vi "Determine Platform.vi"(8 "error in (no error)":errorcluster) -> (0 "error out":errorcluster, 3 "Platform":T1)   [LabVIEW 2020, in "binary_installation_tools.lvlib"]
uses:
  binary_installation_tools.lvlib
  Binary Dependency Platform.ctl
  <vilib>/Utility/error.llb/Clear Errors.vi
  <vilib>/Platform/system.llb/System Exec.vi
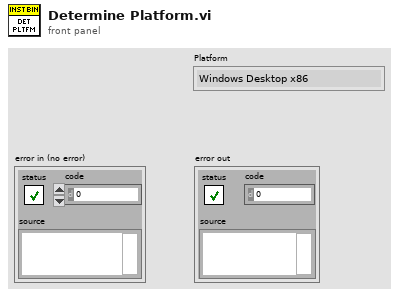
[diagram p1: front panel]
types:
  T1 = typedef "binary_installation_tools.lvlib/Binary Dependency Platform.ctl" = enum16{"Windows Desktop x86", "Windows Desktop x64", "Linux Desktop x64", "Linux Desktop aarch64", "NI Linux RT x64", "NI Linux RT armv7a"}
  T2 = typedef "binary_installation_tools.lvlib/Processor Architecture.ctl" = enum16{"Unknown", "x86", "x64", "arm", "arm64"}
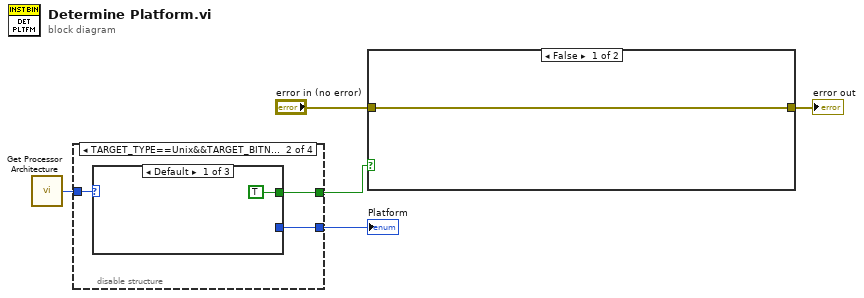
[diagram p0: block diagram]
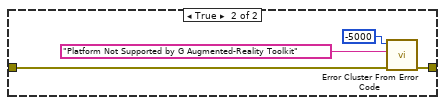
[diagram p2: hidden frame]
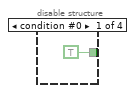
[diagram p3: hidden frame]
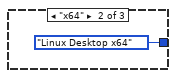
[diagram p4: hidden frame]
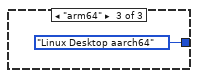
[diagram p5: hidden frame]
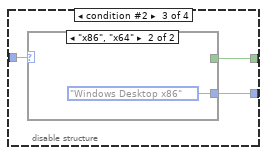
[diagram p6: hidden frame]
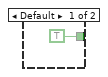
[diagram p7: hidden frame]
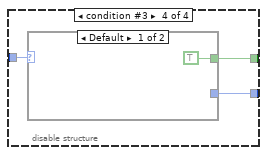
[diagram p8: hidden frame]
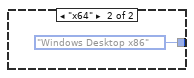
[diagram p9: hidden frame]
diagram:
  n1 = call "Get Processor Architecture.vi"() -> ("Processor Architecture"=w1:T2)
  n2 = disable-structure shown="TARGET_TYPE==Unix&&TARGET_BITNESS==64" {
    disable-tunnel: [_ w9 w15 w20] -> w5
    disable-tunnel: [TRUE w7 w13 w18] -> w2
    disable-tunnel: w1 -> [_ w8 w14 w19]
    frame condition #0 {
    }
    frame condition #1 (active) {
      n3 = case shown="Default" w8 {
        tunnel: [_ Binary_Dependency_Platform."Linux Desktop x64" ("Platform") Binary_Dependency_Platform."Linux Desktop aarch64" ("Platform")] -> w9
        tunnel: [TRUE _ _] -> w7
        frame Default {
        }
        frame "x64" {
        }
        frame "arm64" {
        }
      }
    }
    frame condition #2 {
      n4 = case shown="\"x86\", \"x64\"" w14 {
        tunnel: [_ Binary_Dependency_Platform."Windows Desktop x86" ("Platform")] -> w15
        tunnel: [TRUE _] -> w13
        frame Default {
        }
        frame "x86", "x64" {
        }
      }
    }
    frame condition #3 {
      n5 = case shown="Default" w19 {
        tunnel: [_ Binary_Dependency_Platform."Windows Desktop x86" ("Platform")] -> w20
        tunnel: [TRUE _] -> w18
        frame Default {
        }
        frame "x64" {
        }
      }
    }
  }
  "Platform" <- w5
  n6 = case shown="False" w2 {
    tunnel: "error in (no error)" -> [w23 w27]
    tunnel: [w23 w24] -> w3
    frame False {
    }
    frame True {
      n7 = call <vilib>:"Error Cluster From Error Code.vi"("error in (no error)"=w27, "error message (\"\")"="Platform Not Supported by G Augmented-Reality Toolkit" ("error message (\"\")"), "error code (0)"=-5000) -> ("error out"=w24:errorcluster)  [unwired: 6 in]
    }
  }
  "error out" <- w3
